vi "construct.vi"(6 "cushion_model":T1 items=["Model 1", "Model 2"], 8 "error in (no error)":errorcluster, 9 "cost":dbl, 10 "id":u32) -> (0 "error out":errorcluster, 3 "Chair out":refnum<class "Chair.lvclass">)   [LabVIEW 2021, in "Chair.lvclass"]
uses:
  Chair.lvclass
  IChair/CushionModel.ctl
  Chair.lvclass/Chair.ctl
  IChair/IChair.lvclass
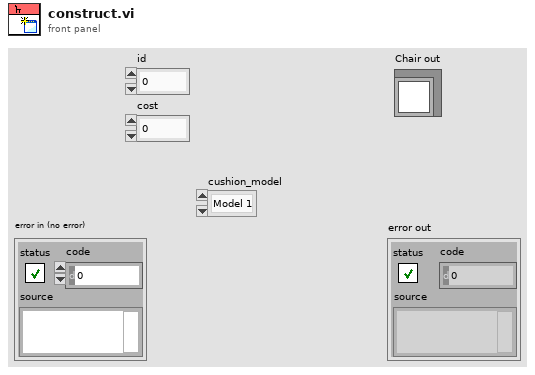
[diagram p1: front panel]
types:
  T1 = typedef "IChair.lvclass/CushionModel.ctl" = u16
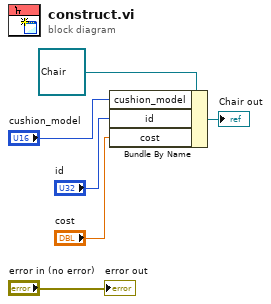
[diagram p0: block diagram]
diagram:
  n1 = Bundle By Name(cluster=refnum<class "Chair.lvclass"> refnum ("Chair.lvclass"), "cushion_model"="cushion_model", "id"="id", "cost"="cost") -> (→"Chair out":refnum<class "Chair.lvclass">)
  "error out" <- "error in (no error)"
